vi "verify_matrices.vi"() -> ()   [LabVIEW 2015]
uses:
  <vilib>/rvi/interface/nirviMethod/nirviMethod.xnode
  <vilib>/rvi/errors/niLvFpgaMergeErrorWithErrorCode.vi
  <vilib>/rvi/interface/nirviReadWriteControl/nirviReadWriteControl.xnode
  <vilib>/FPGAPlugInAG/Dynamic/niLvFpga_Reset_Dynamic.vi
  <vilib>/rvi/interface/nirviOpenFPGA/nirviOpenFPGA.xnode
  <vilib>/rvi/interface/Simulation/niFpgaSimulationCallBeginRW.vi
  <vilib>/rvi/errors/niLvFpgaAdjustHostInterfaceError.vi
  <vilib>/Utility/error.llb/Error Cluster From Error Code.vi
  <vilib>/rvi/interface/nirviCloseFPGA/nirviCloseFPGA.xnode
  <vilib>/FPGAPlugInAG/Dynamic/niLvFpga_Run_Dynamic.vi
  <vilib>/FPGAPlugInAG/Dynamic/niLvFpga_ConfigureFifo_Dynamic.vi
  NiFpgaLv.dll
  <vilib>/FPGAPlugInAG/Dynamic/niLvFpga_WriteFifo_Dynamic.vi
  <vilib>/FPGAPlugInAG/Dynamic/niLvFpga_Close_Dynamic.vi
  FPGA Bitfiles/XYpeizocontrol_FPGATargetSPARTA_testMatrixloadfp_jBmJaQ1o7pM.lvbitx
  fpga_VIs/fpga_UnitTests/testMatrix_load_fpga.vi
  <vilib>/FPGAPlugInAG/cRIO-9082/niLvFpga_Open_cRIO-9082.vi
  <vilib>/rvi/interface/common/dynamic/niFpgaDynamicAddResources.vi
panel:
  out "Ar1":sgl[](array[numeric])
  out "L":sgl[](array[numeric])
  out "Elements Remaing":i32
  in  "NS":i32
  out "All matrix 2":sgl[](array[numeric])
  out "B":sgl[](array[numeric])
  out "Iter":i32
  out "Depth":i32
  in  "Boolean":bool=TRUE
  out "error constant":errorcluster
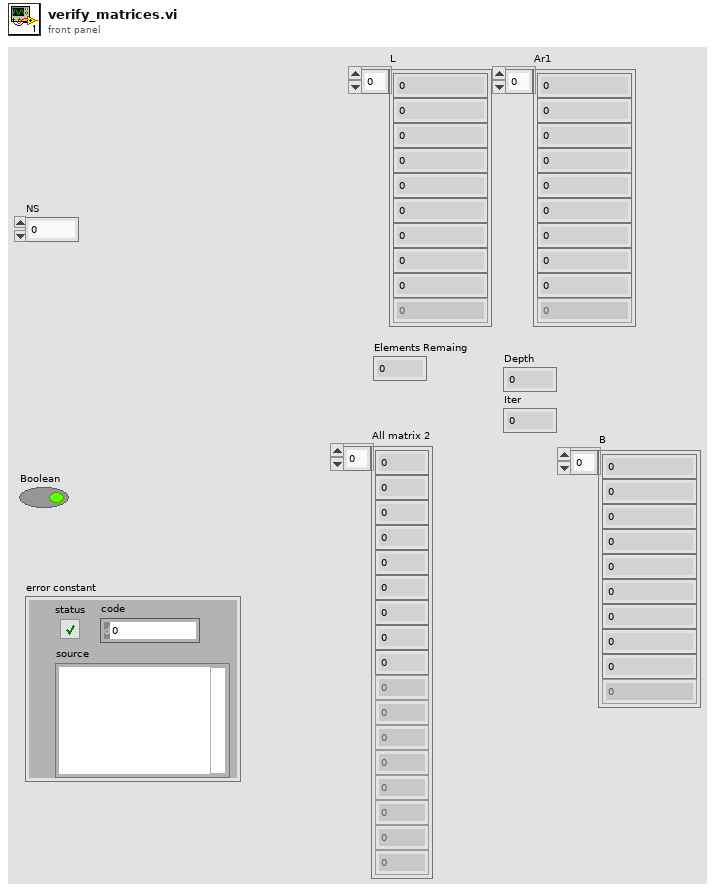
[diagram p1: front panel]
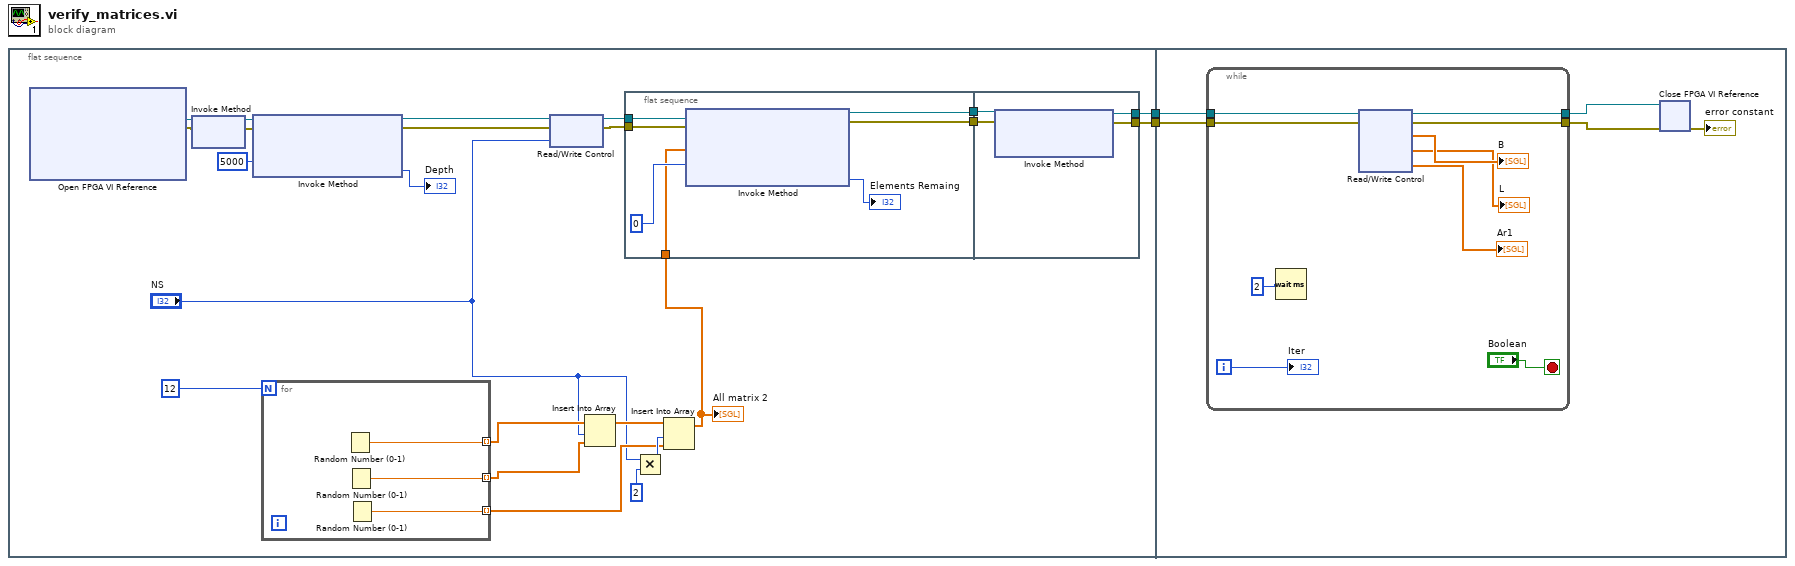
[diagram p0: block diagram]
diagram:
  n1 = flat-sequence {
    tunnel: [w17] -> w2
    tunnel: [w16] -> w1
    tunnel: w2 -> [w43]
    tunnel: w1 -> [w42]
    frame #0 {
      n2 = xnode "Open FPGA VI Reference"() -> ("FPGA VI Reference Out"=w21:refnum<k20>, "error out"=w22:errorcluster)  [unwired: 2 in]
      n3 = xnode "Invoke Method"("FPGA VI Reference In"=w21, "error in"=w22) -> ("FPGA VI Reference Out"=w24:refnum<k20>, "error out"=w25:errorcluster)
      n4 = xnode "Invoke Method"("FPGA VI Reference In"=w24, "error in"=w25, "Requested Depth"=5000) -> ("FPGA VI Reference Out"=w15:refnum<k20>, "error out"=w14:errorcluster, "Actual Depth"=→"Depth":u32)
      n5 = for {
        N: 12 -> [_]
        tunnel: [w28] -> w13 mode=indexing
        tunnel: [w27] -> w12 mode=indexing
        tunnel: [w26] -> w9 mode=indexing
        n6 = Random Number (0-1)() -> (number: 0 to 1=w28:dbl)
        n7 = Random Number (0-1)() -> (number: 0 to 1=w27:dbl)
        n8 = Random Number (0-1)() -> (number: 0 to 1=w26:dbl)
      }
      n9 = xnode "Read/Write Control"("FPGA VI Reference In"=w15, "error in"=w14, "NS"="NS") -> ("FPGA VI Reference Out"=w19:refnum<k20>, "error out"=w18:errorcluster)
      n10 = Insert Into Array(array=w13, index="NS", new element=w12) -> (w11:dbl[])
      n11 = flat-sequence {
        tunnel: w7 -> [w34]
        tunnel: w19 -> [w33]
        tunnel: w18 -> [w32]
        tunnel: [w31] -> w6
        tunnel: [w30] -> w5
        tunnel: w6 -> [w39]
        tunnel: w5 -> [w38]
        tunnel: [w37] -> w17
        tunnel: [w36] -> w16
        frame #0 {
          n12 = xnode "Invoke Method"("FPGA VI Reference In"=w33, "error in"=w32, "Data"=w34, "Timeout (ms)"=0) -> ("FPGA VI Reference Out"=w31:refnum<k20>, "error out"=w30:errorcluster, "Empty Elements Remaining"=→"Elements Remaing":u32)
        }
        frame #1 {
          n13 = xnode "Invoke Method"("FPGA VI Reference In"=w39, "error in"=w38) -> ("FPGA VI Reference Out"=w37:refnum<k20>, "error out"=w36:errorcluster)  [unwired: 1 in]
        }
      }
      n14 = Multiply(x="NS", y=2) -> (x*y=w10:i32)
      n15 = Insert Into Array(array=w11, index=w10, new element=w9) -> (w7:dbl[])
      "All matrix 2" <- w7
    }
    frame #1 {
      n16 = while {
        tunnel: [w48] -> w40
        tunnel: [w47] -> w41
        tunnel: w43 -> [w51]
        tunnel: w42 -> [w50]
        i -> [w54]
        stop <- "Boolean" stop-if-true
        n17 = Wait (ms)(milliseconds to wait=2) -> ()  [unwired: 1 out]
        n18 = xnode "Read/Write Control"("FPGA VI Reference In"=w51, "error in"=w50) -> ("FPGA VI Reference Out"=w48:refnum<k20>, "error out"=w47:errorcluster, "Bz"=→"B":sgl[], "L"=→"L":sgl[], "Arow1"=→"Ar1":sgl[])
        "Iter" <- w54
      }
      n19 = xnode "Close FPGA VI Reference"("FPGA VI Reference In"=w40, "error in"=w41) -> ("error out"=→"error constant":errorcluster)
    }
  }
